vi "Validate Aliases.vi"(8 "error in":errorcluster, 10 "validation information in":T1={"Missing Modules"=variant(cluster{"ID":string, "Path":string}[] []), "Module Connection Map"=variant, "Unused Modules"=variant(cluster{"ID":string, "Path":string}[] [])}, 11 "routing and faulting in":T2 format="%.0x") -> (0 "error out":errorcluster, 1 "aliases errors":errorcluster[](array[cluster]), 2 "validation information out":T1={"Missing Modules"=variant(cluster{"ID":string, "Path":string}[] []), "Module Connection Map"=variant, "Unused Modules"=variant}, 3 "routing and faulting out":T2 format="%.0x")   [LabVIEW 2020, in "Routing and Faulting Scripting.lvlib"]
uses:
  Routing and Faulting Scripting.lvlib
  <vilib>/NI VeriStand/Custom Device API/Custom Device Item Ref.ctl
  Validation Information.ctl
  Shared/Routing and Faulting Hardware API/Routing and Faulting Hardware API.lvlib
  <vilib>/NI VeriStand/Custom Device API/Custom Device API.lvlib
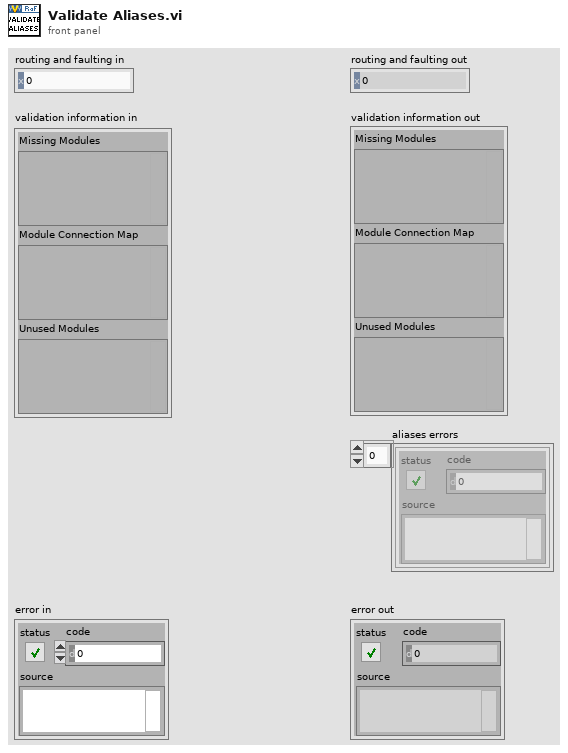
[diagram p1: front panel]
types:
  T1 = typedef "Routing and Faulting Scripting.lvlib/Validation Information.ctl" = cluster{"Missing Modules":variant, "Module Connection Map":variant, "Unused Modules":variant}
  T2 = typedef "Custom Device API.lvlib/Custom Device Item Ref.ctl" = u64
  T3 = typedef "Routing and Faulting Shared.lvlib/Alias Mapping.ctl" = cluster{"Alias":string, "Endpoint":T4}
  T4 = typedef "Routing and Faulting Shared.lvlib/Alias Endpoint.ctl" = cluster{"Module Path":string, "Endpoint":string}
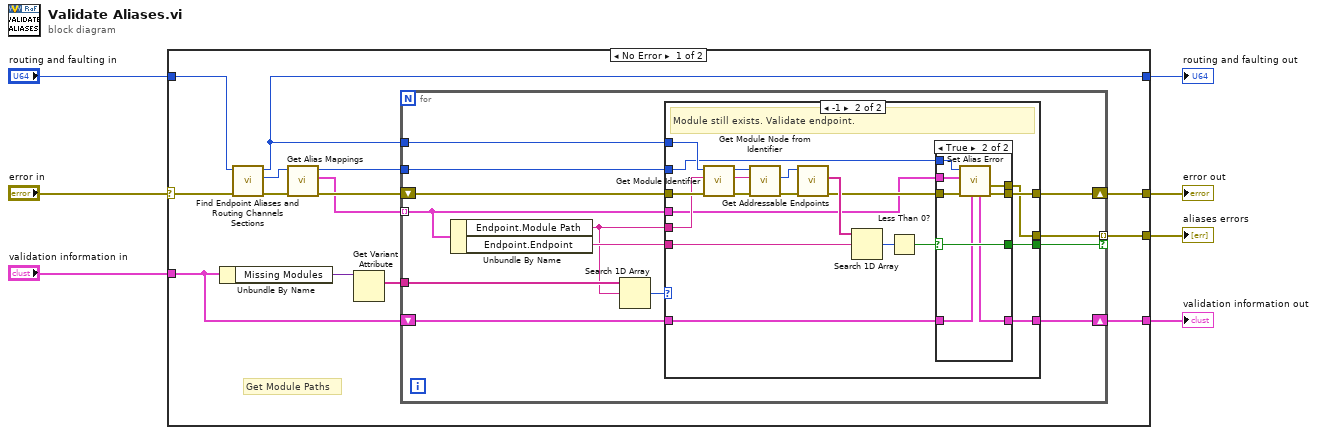
[diagram p0: block diagram]
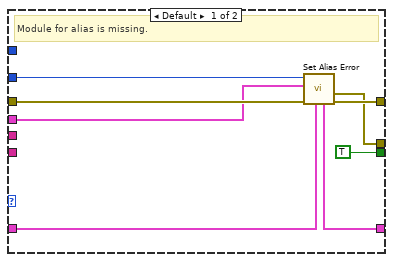
[diagram p2: hidden frame]
diagram:
  n1 = case shown="No Error" "error in" {
    selector: "error in" -> [w14 w76]
    tunnel: "routing and faulting in" -> [w8 w75]
    tunnel: [w17 w76] -> w6
    tunnel: [w13 w75] -> w5
    tunnel: [w15 _] -> w4
    tunnel: "validation information in" -> [w12 w74]
    tunnel: [w11 w74] -> w1
    frame No Error {
      # "Get Module Paths"
      n2 = Unbundle By Name(w12) -> ("Missing Modules"=w10:variant)
      n3 = call "Find Endpoint Aliases and Routing Channels Sections.vi"("error in"=w14, "routing and faulting custom device in"=w8) -> ("error out"=w21:errorcluster, "endpoint aliases"=w20:T2, "routing and faulting custom device out"=w13:T2)  [unwired: 6 in, 1 out]
      n4 = call "Get Alias Mappings.vi"("error in"=w21, "endpoint aliases in"=w20) -> ("error out"=w19:errorcluster, "alias mappings"=w16:T3[], "endpoint aliases out"=w18:T2)  [unwired: 7 in]
      n5 = Get Variant Attribute(Variant=w10) -> (names=w9:string[])  [unwired: 3 in, 3 out]
      n6 = for {
        tunnel: w16 -> [w26] mode=indexing
        tunnel: w9 -> [w34]
        shift-right: [w31] -> w17
        shift-left: w19 -> [w32]
        tunnel: [w30] -> w15 mode=indexing if=w25
        tunnel: w13 -> [w27]
        tunnel: w18 -> [w29]
        shift-right: [w22] -> w11
        shift-left: w12 -> [w23]
        n7 = Unbundle By Name(w26) -> ("Endpoint.Module Path"=w24:string, "Endpoint.Endpoint"=w28:string)
        n8 = Search 1D Array(1D array=w34, element=w24) -> (index of element=w33:i32)  [unwired: 1 in]
        n9 = case shown="-1" w33 {
          tunnel: w32 -> [w41 w62]
          tunnel: [w40 w49] -> w31
          tunnel: [TRUE w45] -> w25
          tunnel: w24 -> [_ w61]
          tunnel: [w39 w48] -> w30
          tunnel: w29 -> [w38 w46]
          tunnel: w28 -> [_ w53]
          tunnel: w27 -> [_ w52]
          tunnel: w26 -> [w37 w47]
          tunnel: w23 -> [w36 w44]
          tunnel: [w35 w43] -> w22
          frame Default {
            # "Module for alias is missing."
            n10 = call "Set Alias Error.vi"("validation information in"=w36, "error in"=w41, "alias"=w37, "endpoint aliases in"=w38) -> ("error out"=w40:errorcluster, "veristand error out"=w39:errorcluster, "validation information out"=w35:T1)  [unwired: 4 in, 1 out]
          }
          frame -1 {
            # "Module still exists. Validate endpoint."
            n11 = call "Get Module Identifier.vi"("error in"=w62, "module path"=w61, "routing and faulting in"=w52) -> ("error out"=w60:errorcluster, "module identifier"=w58:string, "routing and faulting out"=w59:T2)  [unwired: 5 in, 1 out]
            n12 = call "Get Module Node from Identifier.vi"("error in"=w60, "module identifier"=w58, "routing and faulting in"=w59) -> ("error out"=w57:errorcluster, "module node"=w56:T2)  [unwired: 5 in, 2 out]
            n13 = call "Get Addressable Endpoints.vi"("error in (no error)"=w57, "Hardware Ref in"=w56) -> ("error out"=w51:errorcluster, "Addressable Endpoints"=w55:string[])  [unwired: 6 in, 2 out]
            n14 = Search 1D Array(1D array=w55, element=w53) -> (index of element=w54:i32)  [unwired: 1 in]
            n15 = Less Than 0?(x=w54) -> (x < 0?=w50:bool)
            n16 = case shown="True" w50 {
              selector: w50 -> [w63 w68]
              tunnel: w51 -> [w65 w73]
              tunnel: [w65 w72] -> w49
              tunnel: [_ w71] -> w48
              tunnel: w47 -> [_ w70]
              tunnel: w46 -> [_ w69]
              tunnel: [w63 w68] -> w45
              tunnel: w44 -> [w64 w67]
              tunnel: [w64 w66] -> w43
              frame False {
              }
              frame True {
                n17 = call "Set Alias Error.vi"("validation information in"=w67, "error in"=w73, "alias"=w70, "endpoint aliases in"=w69) -> ("error out"=w72:errorcluster, "veristand error out"=w71:errorcluster, "validation information out"=w66:T1)  [unwired: 4 in, 1 out]
              }
            }
          }
        }
      }
    }
    frame Error {
    }
  }
  "routing and faulting out" <- w5
  "error out" <- w6
  "aliases errors" <- w4
  "validation information out" <- w1
